vi "Global.vi"() -> ()   [LabVIEW 2014]
uses:
  Controls/OtherSpec.ctl
  <vilib>/userdefined/High Color/IMAQdx.ctl
  ModelEditSubVIs/ModeEditeControl.ctl
  ModelEditSubVIs/ModelInfo.ctl
  Controls/XYPos.ctl
panel:
  in  "选项卡控件":enum32{"规格", "路径", "对位时信息"}(tab)
  in  "登陆状态":cluster{"用户名称":string, "用户权限":string}
  in  "其它规格":T1={"其它勾选类规格"={"保存图片"=TRUE, "上传设备状态数据"=TRUE, "保存数据"=TRUE, "开机默认开启监控摄像头"=FALSE, "启用mark拍照 "=FALSE}, "其它数据类规格"={"相机1像素-毫米换算系数"=0.0115, "相机2像素-毫米换算系数"=0.0115, "D盘剩余空间预警(G)"=20.0, "视频最长录制时间(秒)"=600.0}, "相机名称"={"相机1名称"="cam0", "相机2名称"="cam1", "Cam1启用"=TRUE, "Cam2启用"=TRUE, "Basler1"=FALSE, "Basler2"=FALSE}, "参数"={"Mark1曝光时间"=500, "Mark2曝光时间"=500, "二维码曝光时间"=500}} {"其它数据类规格"."视频最长录制时间(秒)" format="%.3f"; "其它数据类规格"."D盘剩余空间预警(G)" format="%.3f"; "其它数据类规格"."相机1像素-毫米换算系数" format="%.5f"; "其它数据类规格"."相机2像素-毫米换算系数" format="%.5f"}
  out "已输入密码":bool
  out "mark Angle":dbl
  out "mark1偏移":T6 {"X" format="%#.3f"}
  in  "补偿值":T8={"甩线补偿值"={"下边"=23.0, "距离上边"=10.0, "左边"=7.2, "右边"=25.8}, "补偿甩线坐标偏移"={"X"=40.0, "Y"=70.0}, "mark点模组补偿"={"X"=-48.38, "Y"=-84.85}, "出线补偿值"=25.8, "mark规格"={"X下限"=-48.38, "X上限"=-84.85, "Y下限"=0.0, "Y 上限"=0.0, "angle下限"=0.0, "angle上限"=0.0}} {"mark规格"."angle上限" format="%#.3f"; "mark规格"."angle下限" format="%#.3f"; "mark规格"."Y下限" format="%#.3f"; "mark规格"."X下限" format="%#.3f"; "mark点模组补偿"."X" format="%#.3f"; "补偿甩线坐标偏移"."X" format="%#.3f"}
  in  "mark 点理论坐标":T9={"mark 1 "={"X"=1.0, "Y"=1.0}, "mark 2"={"X"=1.0, "Y"=1.0}} {"mark 2"."X" format="%#.3f"; "mark 1"."X" format="%#.3f"}
  in  "校准图片路径":path
  out "ModelEditInfo":T10
  in  "批次号":string
  in  "数据保存表格模板":path
  in  "测试图片保存根目录":path
  in  "生产统计根目录":path
  in  "BathPath":path
  in  "测试数据保存根目录":path
  out "夹螺杆：拍照右边螺帽点到取料点dtXY":T6 {"X" format="%#.3f"}
  out "校准1：拍照PCB孔点到放料点距离dtXY补偿":T6 {"X" format="%#.3f"}
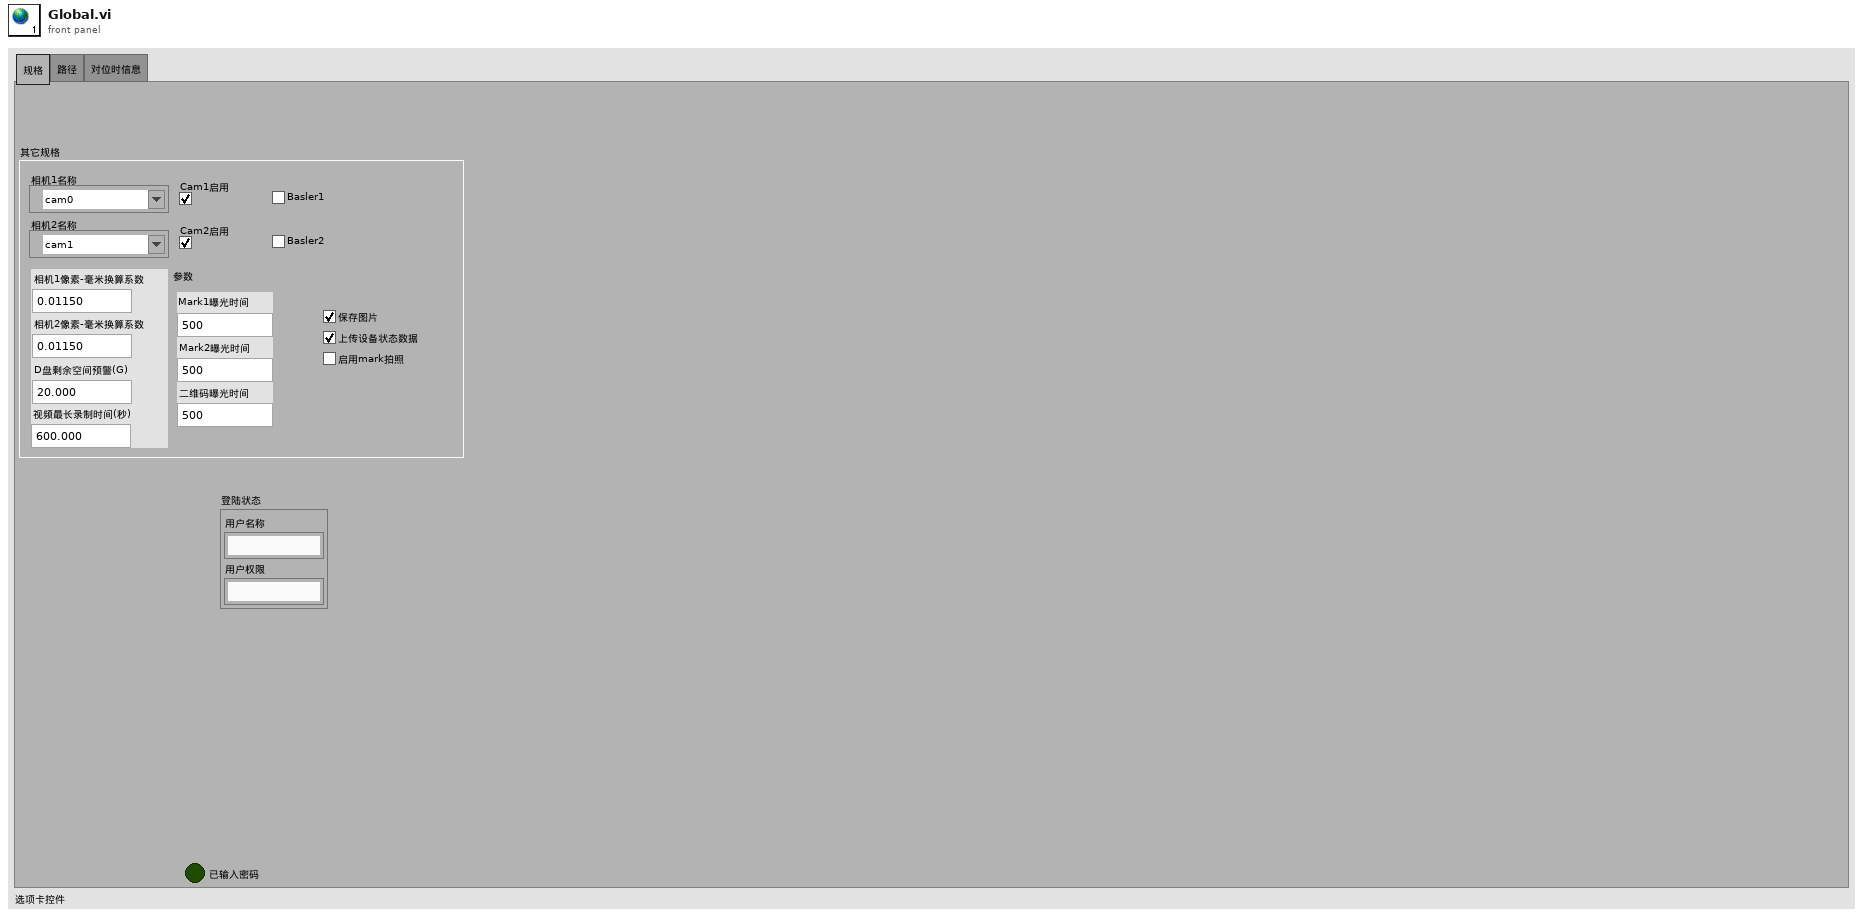
[diagram p1: front panel]
types:
  T1 = typedef "OtherSpec.ctl" = cluster{"其它勾选类规格":T2, "其它数据类规格":T3, "相机名称":T4, "参数":cluster{"Mark1曝光时间":i32, "Mark2曝光时间":i32, "二维码曝光时间":i32}}
  T2 = typedef "其它勾选类规格.ctl" = cluster{"保存图片":bool, "上传设备状态数据":bool, "保存数据":bool, "开机默认开启监控摄像头":bool, "启用mark拍照 ":bool}
  T3 = typedef "其他数据类规格.ctl" = cluster{"相机1像素-毫米换算系数":dbl, "相机2像素-毫米换算系数":dbl, "D盘剩余空间预警(G)":dbl, "视频最长录制时间(秒)":dbl}
  T4 = typedef "相机名称品牌使用状态.ctl" = cluster{"相机1名称":T5, "相机2名称":T5, "Cam1启用":bool, "Cam2启用":bool, "Basler1":bool, "Basler2":bool}
  T5 = typedef "IMAQdx.ctl" = refnum<k21>
  T6 = typedef "XYPos.ctl" = cluster{"X":dbl, "Y":dbl}
  T7 = typedef "mark规格.ctl" = cluster{"X下限":dbl, "X上限":dbl, "Y下限":dbl, "Y 上限":dbl, "angle下限":dbl, "angle上限":dbl}
  T8 = cluster{"甩线补偿值":cluster{"下边":dbl, "距离上边":dbl, "左边":dbl, "右边":dbl}, "补偿甩线坐标偏移":T6, "mark点模组补偿":T6, "出线补偿值":dbl, "mark规格":T7}
  T9 = cluster{"mark 1 ":cluster{"X":dbl, "Y":dbl}, "mark 2":cluster{"X":dbl, "Y":dbl}}
  T10 = typedef "ModeEditeControl.ctl" = cluster{"AllModelFold":path, "AllModelNamePath":path, "所有零件型号":string[], "当前零件型号":string, "所有建立零件信息":string[][], "当前零件序号":i32, "当前产品信息":T11}
  T11 = typedef "ModelInfo.ctl" = cluster{"产品型号":string, "二维码拍照":u32, "Mark点拍照":u32}
diagram:
